vi "Global_Signal.vi"() -> ()   [LabVIEW 2018]
panel:
  out "Signal":dbl[](graph)
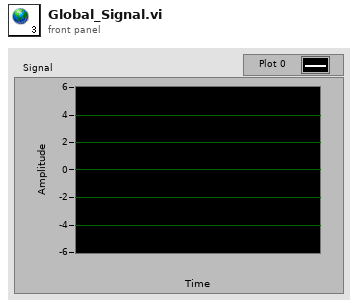
[diagram p1: front panel]
diagram:
